vi "TempDataGraph.vi"() -> ()   [LabVIEW 2020]
panel:
  out "온도 인덱스":u32
  out "XY Graph":cluster{"Y":dbl[], "Y":dbl[]}[](graph) caption="XY 그래프"
  in  "거리해상도":string(combo)="5" caption="거리 해상도"
  out "온도파일문자열":string caption="안티스톡스 파일"
  in  "종료":bool
  in  "다음 데이터":bool
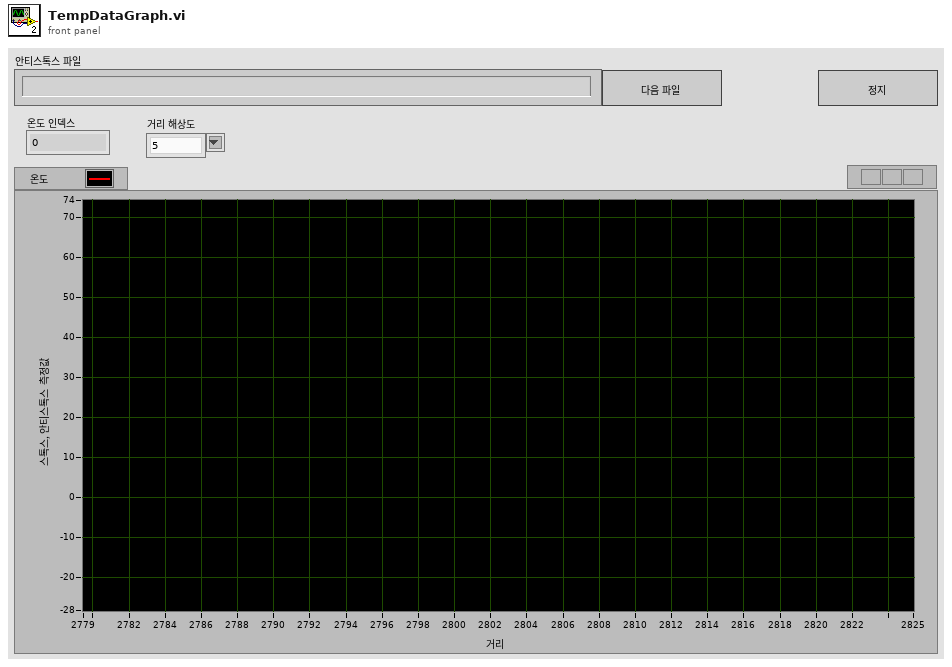
[diagram p1: front panel]
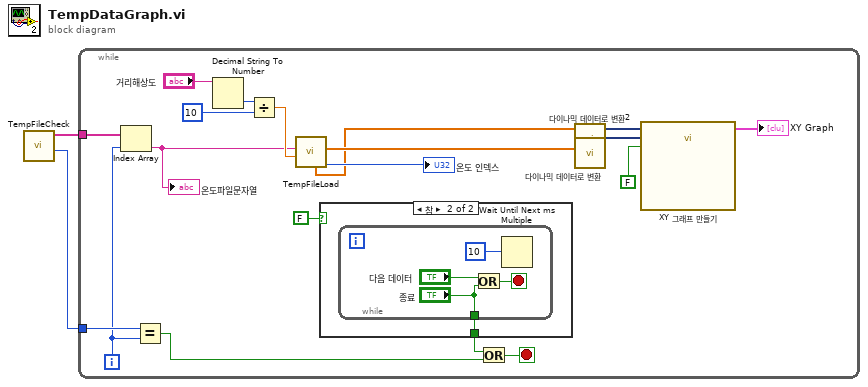
[diagram p0: block diagram]
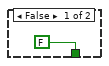
[diagram p2: hidden frame]
diagram:
  n1 = call "TempFileCheck.vi"() -> ("파일수"=w1:u16, "온도 파일 배열"=w2:string[])  [unwired: 9 in, 1 out]
  n2 = while {
    tunnel: w2 -> [w21]
    tunnel: w1 -> [w20]
    i -> [w16]
    stop <- w10 stop-if-true
    n3 = Index Array(array=w21, index=w16) -> (element=w8:string)
    "온도파일문자열" <- w8
    n4 = Equal?(x=w20, y=w16) -> (x = y?=w11:bool)
    n5 = Decimal String To Number(string="거리해상도") -> (number=w15:i32)  [unwired: 2 in, 1 out]
    n6 = Divide(x=w15, y=10) -> (x/y=w13:dbl)
    n7 = call "TempFileLoad.vi"("거리 해상도"=w13, "온도 데이터 경로 문자열"=w8) -> ("온도 인덱스"=→"온도 인덱스":i32, "온도 배열"=w7:dbl[], "거리축 배열"=w5:dbl[])  [unwired: 6 in, 1 out]
    n8 = case shown="참" FALSE {
      tunnel: [FALSE w23] -> w12
      frame False {
      }
      frame True {
        n9 = while {
          tunnel: ["종료"] -> w23
          stop <- w25 stop-if-true
          n10 = Or(x="다음 데이터", y="종료") -> (x .or. y?=w25:bool)
          n11 = Wait Until Next ms Multiple(millisecond multiple=10) -> ()  [unwired: 1 out]
        }
      }
    }
    n12 = Or(x=w12, y=w11) -> (x .or. y?=w10:bool)
    n13 = call "다이나믹 데이터로 변환2"("Array"=w5) -> ("Dynamic Data Type"=w4:dynamicdata)  [unwired: 3 in]
    n14 = call "다이나믹 데이터로 변환"("Array"=w7) -> ("Dynamic Data Type"=w6:dynamicdata)  [unwired: 3 in]
    n15 = call "XY 그래프 만들기"("Reset"=FALSE, "Y Input"=w6, "X Input"=w4) -> ("XY Graph"=→"XY Graph":cluster{"X":dbl[], "Y":dbl[]}[])  [unwired: 7 in, 1 out]
  }
